vi "Main_004.vi"() -> ()   [LabVIEW 2025]
uses:
  Utility/Universal Utility/TypeDefs_Utility/Cluster_Row-Column.ctl
  9e3f57c0-2ef8-4495-8287-c6a42a5fb955.vi
  Utility/Universal Utility/TypeDefs_Utility/ENUM_4 Directions U-D-L-R.ctl
  Utility/Universal Utility/TypeDefs_Utility/ENUM_8 Directions U-D-L-R.ctl
panel:
  out "Numeric":u64
  out "x+y":u64
  out "MATCH":bool
  in  "Select Data":enum32{"Example", "Puzzle"}(tab)
  in  "EX Target":u64=9009
  in  "EX Digits":u64
  in  "Puzzle Digits":u64=3
  in  "Puzzle Target":u64=906609
  out "Answer":u64
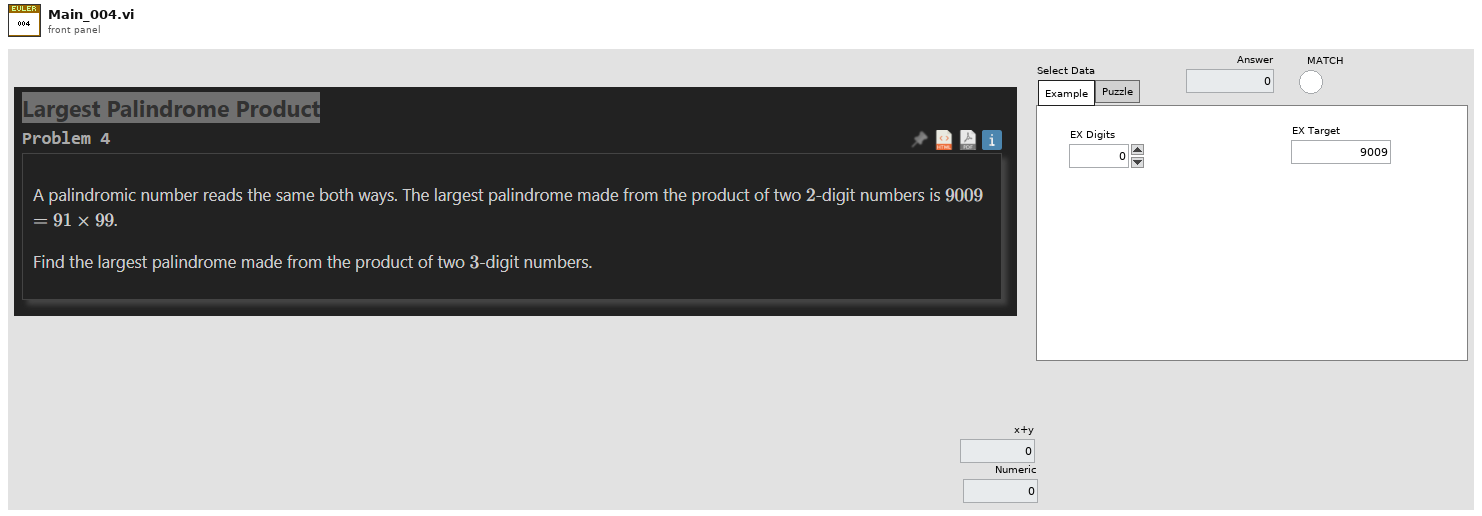
[diagram p1: front panel]
types:
  T1 = typedef "ENUM_8 Directions U-D-L-R.ctl" = enum16{"Up;-1,0", "Up-Right;-1,1", "Right;0,1", "Down-Right;1,1", "Down;1,0", "Down-Left;1,-1", "Left;0,-1", "Up-Left;-1,-1"}
  T2 = typedef "ENUM_4 Directions U-D-L-R.ctl" = enum16{"Up;-1,0", "Right;0,1", "Down;1,0", "Left;0,-1"}
  T3 = typedef "Cluster_Row-Column.ctl" = cluster{"R":i32, "C":i32}
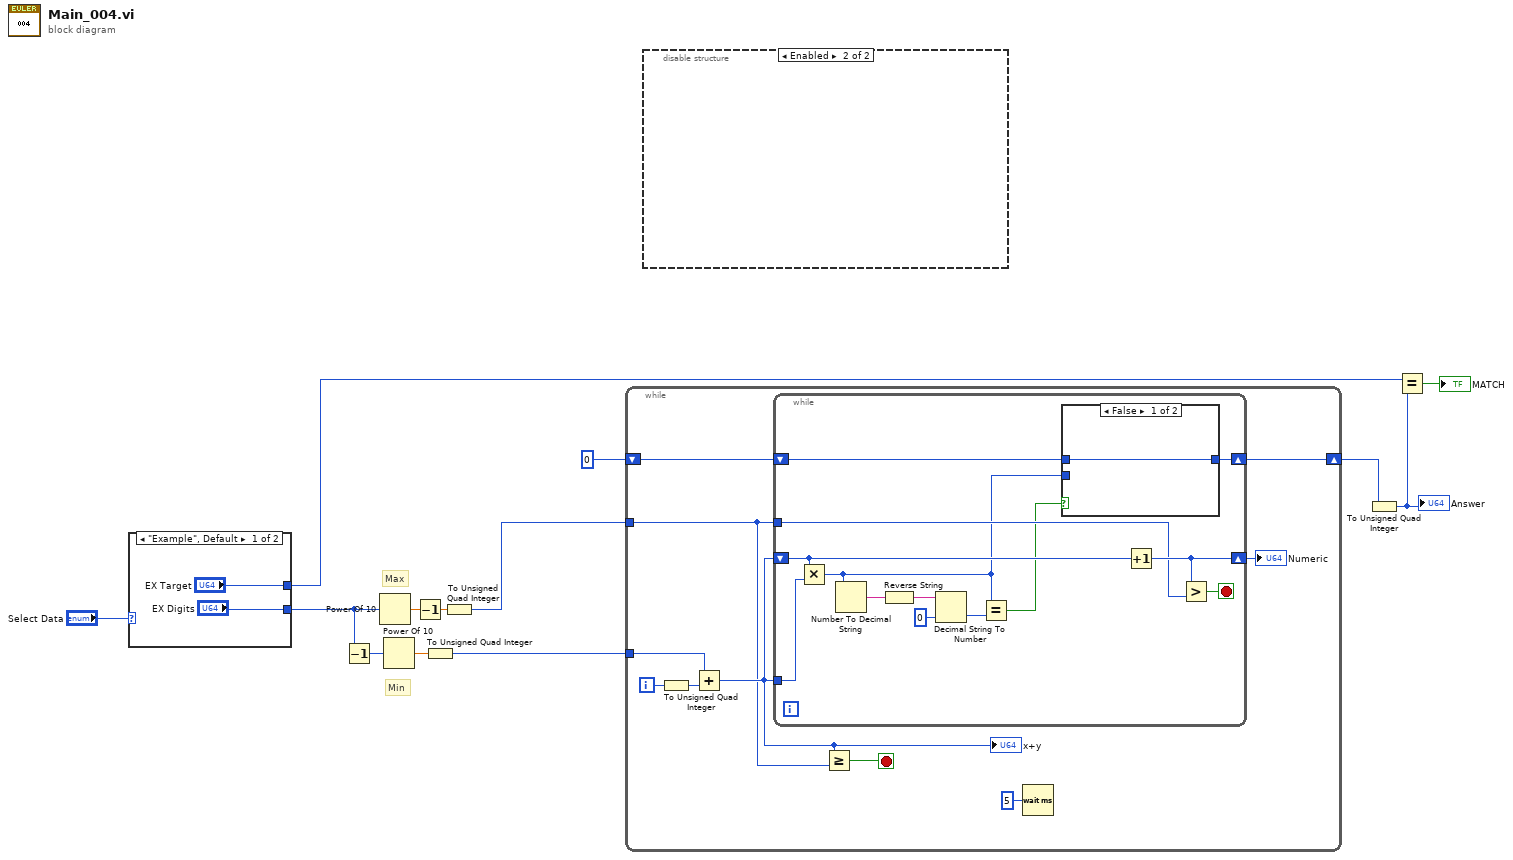
[diagram p0: block diagram]
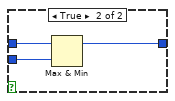
[diagram p2: hidden frame]
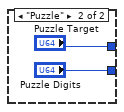
[diagram p3: hidden frame]
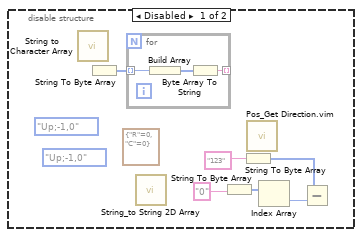
[diagram p4: hidden frame]
diagram:
  # "Min"
  # "Max"
  n1 = case shown="\"Example\", Default" "Select Data" {
    tunnel: ["EX Digits" "Puzzle Digits"] -> w7
    tunnel: ["EX Target" "Puzzle Target"] -> w11
    frame "Example", Default {
    }
    frame "Puzzle" {
    }
  }
  n2 = Decrement(x=w7) -> (x-1=w6:u64)
  n3 = Power Of 10(x=w7) -> (10^x=w9:dbl)
  n4 = Power Of 10(x=w6) -> (10^x=w5:dbl)
  n5 = Decrement(x=w9) -> (x-1=w8:dbl)
  n6 = To Unsigned Quad Integer(1:w5) -> (0:w3:u64)
  n7 = To Unsigned Quad Integer(1:w8) -> (0:w4:u64)
  n8 = while {
    tunnel: w4 -> [w23]
    tunnel: w3 -> [w21]
    shift-right: [w18] -> w1
    shift-left: u64 0 ("unsigned 64bit integer") -> [w19]
    i -> [w26]
    stop <- w25 stop-if-true
    n9 = To Unsigned Quad Integer(1:w26) -> (0:w27:u64)
    n10 = Add(x=w21, y=w27) -> (x+y=w24:u64)
    "x+y" <- w24
    n11 = while {
      shift-right: [w34] -> w20
      shift-left: w24 -> [w35]
      tunnel: w23 -> [w33]
      tunnel: w24 -> [w40]
      shift-right: [w28] -> w18
      shift-left: w19 -> [w30]
      stop <- w32 stop-if-true
      n12 = Multiply(x=w35, y=w40) -> (x*y=w29:u64)
      n13 = Number To Decimal String(number=w29) -> (decimal integer string=w39:string)  [unwired: 1 in]
      n14 = Reverse String(1:w39) -> (0:w38:string)
      n15 = Decimal String To Number(string=w38, default (0L)=u64 0 ("default (0 I32)")) -> (number=w37:u64)  [unwired: 1 in, 1 out]
      n16 = Equal?(x=w29, y=w37) -> (x = y?=w31:bool)
      n17 = case shown="False" w31 {
        tunnel: w30 -> [w41 w44]
        tunnel: w29 -> [_ w43]
        tunnel: [w41 w42] -> w28
        frame False {
        }
        frame True {
          n18 = Max & Min(x=w44, y=w43) -> (max(x,y)=w42:u64)  [unwired: 1 out]
        }
      }
      n19 = Increment(x=w35) -> (x+1=w34:u64)
      n20 = Greater?(x=w34, y=w33) -> (0:w32:bool)
    }
    "Numeric" <- w20
    n21 = Greater Or Equal?(x=w24, y=w23) -> (x >= y?=w25:bool)
    n22 = Wait (ms)(milliseconds to wait=u32 5) -> ()  [unwired: 1 out]
  }
  n23 = disable-structure shown="Enabled" {
    frame Disabled {
      (unwired) ENUM_8_Directions_U-D-L-R."Up;-1,0" ("Direction 8")
      (unwired) ENUM_4_Directions_U-D-L-R."Up;-1,0" ("Direction")
      (unwired) T3 {"R"=0, "C"=0} ("Position")
      n24 = call "String to Character Array.vi"() -> ()  [unwired: 1 in, 1 out]
      n25 = String To Byte Array() -> (unsigned byte array=w45:u8[])  [unwired: 1 in]
      n26 = for {
        tunnel: w45 -> [w53] mode=indexing
        tunnel: [w51] -> _ mode=indexing
        n27 = Build Array(w53) -> (w52:u8[])
        n28 = Byte Array To String(unsigned byte array=w52) -> (string=w51:string)
      }
      n29 = call "String_to String 2D Array.vi"() -> ()  [unwired: 11 in, 1 out]
      n30 = String To Byte Array(string="0") -> (unsigned byte array=w48:u8[])
      n31 = String To Byte Array(string="123") -> (unsigned byte array=w46:u8[])
      n32 = call "Pos_Get Direction.vim"() -> ()  [unwired: 11 in, 1 out]
      n33 = Index Array(array=w48) -> (element=w47:u8)  [unwired: 1 in]
      n34 = Subtract(x=w46, y=w47) -> ()  [unwired: 1 out]
    }
    frame Enabled {
    }
  }
  n35 = To Unsigned Quad Integer(1:w1) -> (0:w10:u64)
  "Answer" <- w10
  n36 = Equal?(x=w11, y=w10) -> (x = y?=→"MATCH":bool)
